vi "reverse data if odd index.vi"(10 "Scan Index":i32, 11 "In":dbl[][](array[numeric])) -> (3 "Out":dbl[][](array[numeric]))   [LabVIEW 2014]
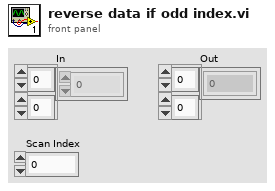
[diagram p1: front panel]
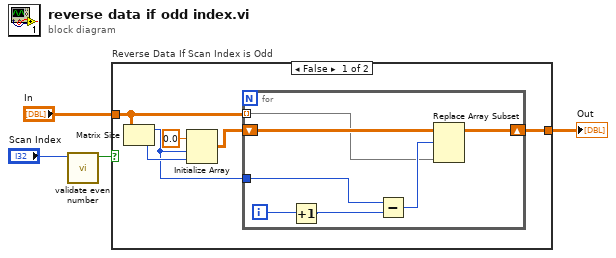
[diagram p0: block diagram]
diagram:
  n1 = call "validate even number.vi"("Number"="Scan Index") -> ("Even"=w2:bool)  [unwired: 10 in]
  n2 = case "Reverse Data If Scan Index is Odd" shown="False" w2 {
    tunnel: "In" -> [w8 w18]
    tunnel: [w6 w18] -> w4
    frame False {
      n3 = Matrix Size(0:w8) -> (1:w5:i32, 2:w10:i32)
      n4 = Initialize Array(0.0 ("element"), w5, w10) -> (w7:dbl[][])
      n5 = for {
        tunnel: w8 -> [w14] mode=indexing
        shift-right: [w16] -> w6
        shift-left: w7 -> [w17]
        tunnel: w5 -> [w13]
        i -> [w12]
        n6 = Increment(x=w12) -> (x+1=w11:i32)
        n7 = Subtract(x=w13, y=w11) -> (x-y=w15:i32)
        n8 = Replace Array Subset(array=w17, new element=w14, index (row)=w15) -> (w16:dbl[][])  [unwired: 1 in]
      }
    }
    frame True {
    }
  }
  "Out" <- w4
